vi "随机数发生器（Wishmann-Hill均匀分布）.vi"(0 "Seed":i32, 1 "Reset":bool) -> (4 "Ui":dbl)   [LabVIEW 2012]
doc: "功能：\n\n产生0-32768之间的随机整数。\n\n基本算法：\n\n使用同乘余法。\n\ncsxcs_366创建"
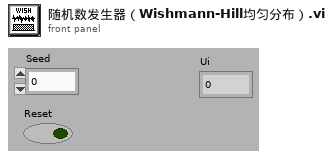
[diagram p1: front panel]
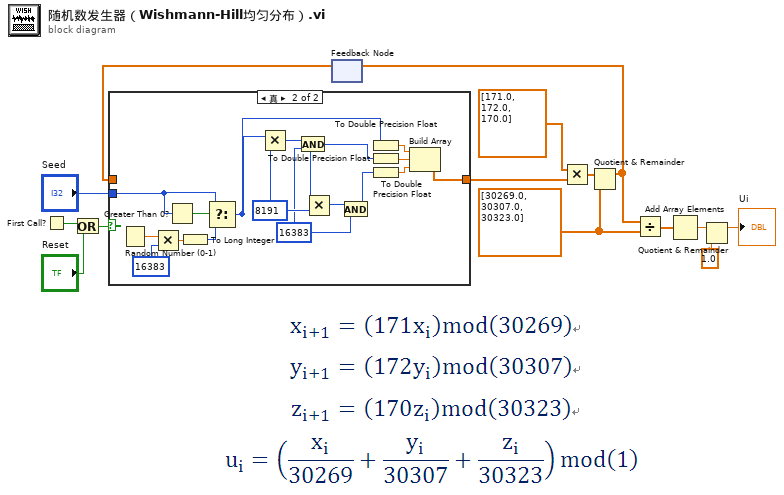
[diagram p0: block diagram]
diagram:
  w6 = dbl[] [30269.0, 30307.0, 30323.0]
  n1 = First Call?() -> (First Call?: T/F=w14:bool)
  n2 = Or(x=w14, y="Reset") -> (x .or. y?=w12:bool)
  n3 = feedback #1() -> (w11:dbl[])  [unwired: 1 in]
  n4 = case shown="真" w12 {
    tunnel: w11 -> [w15 _]
    tunnel: [w15 w17] -> w9
    tunnel: "Seed" -> [_ w16]
    frame False {
    }
    frame True {
      w25 = 16383
      w27 = 8191 ("y")
      n5 = Random Number (0-1)() -> (number: 0 to 1=w30:dbl)
      n6 = Multiply(x=w30, y=16383 ("x")) -> (x*y=w29:dbl)
      n7 = Greater Than 0?(x=w16) -> (x > 0?=w28:bool)
      n8 = To Long Integer(number=w29) -> (32bit integer=w32:i32)
      n9 = Select(t=w16, s=w28, f=w32) -> (s? t:f=w23:i32)
      n10 = Multiply(x=w23, y=w27) -> (x*y=w24:i32)
      n11 = And(x=w24, y=w25) -> (x .and. y?=w22:i32)
      n12 = Multiply(x=w22, y=w27) -> (x*y=w26:i32)
      n13 = And(x=w25, y=w26) -> (x .and. y?=w21:i32)
      n14 = To Double Precision Float(number=w23) -> (double precision float=w19:dbl)
      n15 = To Double Precision Float(number=w22) -> (double precision float=w20:dbl)
      n16 = To Double Precision Float(number=w21) -> (double precision float=w18:dbl)
      n17 = Build Array(w19, w20, w18) -> (w17:dbl[])
    }
  }
  n18 = Multiply(x=dbl[] [171.0, 172.0, 170.0], y=w9) -> (x*y=w8:dbl[])
  n19 = Quotient & Remainder(x=w8, y=w6) -> (x-y*floor(x/y)=w7:dbl[])  [unwired: 1 out]
  n20 = feedback-in #1(w7) -> ()
  n21 = Divide(x=w7, y=w6) -> (x/y=w5:dbl[])
  n22 = Add Array Elements(numeric array=w5) -> (sum=w4:dbl)
  n23 = Quotient & Remainder(x=w4, y=1.0) -> (x-y*floor(x/y)=→"Ui":dbl)  [unwired: 1 out]
